vi "Get Project Application Instance.vi"(8 "error in (no error)":errorcluster) -> (0 "error out":errorcluster, 3 "Application out":refnum<vi>)   [LabVIEW 2020, in "Method Generation.lvlib" / "Setter Generator.lvclass"]
uses:
  Setter Generator.lvclass
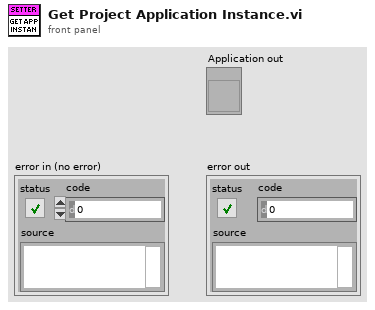
[diagram p1: front panel]
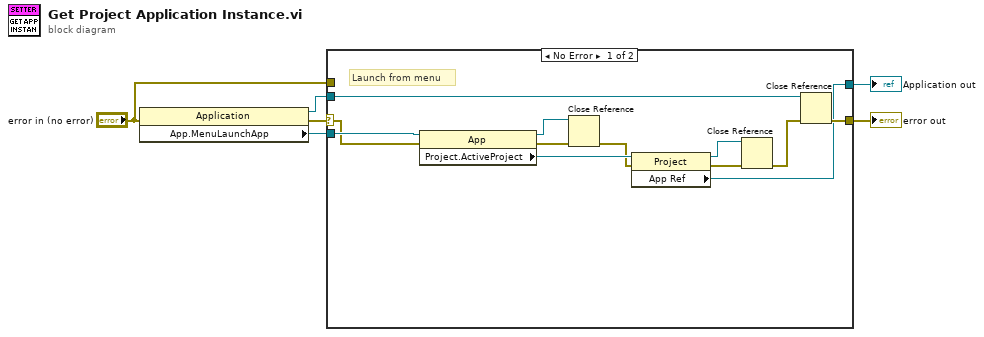
[diagram p0: block diagram]
diagram:
  n1 = property class="Application"(error in="error in (no error)") -> (reference out=w3:refnum<vi>, error out=w2:errorcluster, "App.MenuLaunchApp"=w1:refnum<vi>)  [unwired: 1 in]
  n2 = case shown="No Error" w2 {
    selector: w2 -> [w8 _]
    tunnel: [w14 w20] -> w5
    tunnel: w1 -> [w15 _]
    tunnel: [w17 w19] -> w6
    tunnel: "error in (no error)" -> [_ w19]
    tunnel: w3 -> [w18 w20]
    frame No Error {
      # "Launch from menu"
      n3 = property class="App"(reference=w15, error in=w8) -> (reference out=w10:refnum<vi>, error out=w11:errorcluster, "Project.ActiveProject"=w16:refnum<vi>)
      n4 = Close Reference(reference=w10, error in (no error)=w11) -> (error out=w9:errorcluster)
      n5 = property class="Project"(reference=w16, error in=w9) -> (reference out=w13:refnum<vi>, error out=w12:errorcluster, "App Ref"=w14:refnum<vi>)
      n6 = Close Reference(reference=w13, error in (no error)=w12) -> (error out=w7:errorcluster)
      n7 = Close Reference(reference=w18, error in (no error)=w7) -> (error out=w17:errorcluster)
    }
    frame Error {
    }
  }
  "error out" <- w6
  "Application out" <- w5
